vi "Set Serial Settings.vi"(8 "error in (no error)":errorcluster, 11 "LED in":refnum<class "LED.lvclass">) -> (0 "error out":errorcluster, 3 "LED out":refnum<class "LED.lvclass">)   [LabVIEW 2016, in "LED.lvclass"]
uses:
  LED.lvclass
  Desktop/platinum-modbus-driver/omega_engineering-platinum-modbus-driver-671bd10261c3/Labview Source Code/Platinum Serial Modbus/Platinum_MB_SerHandle.ctl
  Desktop/platinum-modbus-driver/omega_engineering-platinum-modbus-driver-671bd10261c3/Labview Source Code/Platinum Serial Modbus/Platinum_MB_serMode.ctl
  Desktop/platinum-modbus-driver/omega_engineering-platinum-modbus-driver-671bd10261c3/Labview Source Code/Platinum Serial Modbus/Platinum_MB_serFlowControl.ctl
  Desktop/platinum-modbus-driver/omega_engineering-platinum-modbus-driver-671bd10261c3/Labview Source Code/Platinum Serial Modbus/Platinum_MB_serParity.ctl
  LED.lvclass/LED.ctl
  LightBox/LightBox.lvclass
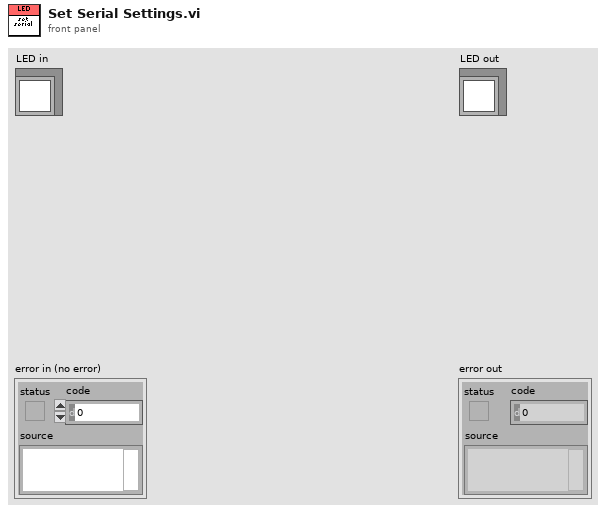
[diagram p1: front panel]
types:
  T1 = typedef "Platinum_MB_serFlowControl.ctl" = enum16{"None", "XON_XOFF", "RTS_CTS", "XON_XOFF_and_RTS_CTS", "DTR_DSR", "XON_XOFF_and_DTR_DSR"}
  T2 = typedef "Platinum_MB_serMode.ctl" = enum16{"RTU", "ASCII"}
  T3 = typedef "Platinum_MB_serParity.ctl" = enum16{"None", "Odd", "Even", "Mark", "Space"}
  T4 = typedef "Platinum_MB_SerHandle.ctl" = cluster{"VISAResourceName":string, "Mode":T2, "Timeout":u32, "FlowControl":T1, "Parity":T3, "BaudRate":u32, "SlaveAddress":u8}
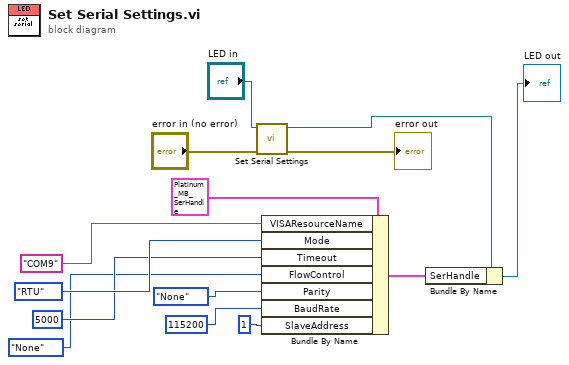
[diagram p0: block diagram]
diagram:
  n1 = call-parent "Set Serial Settings.vi"("error in (no error)"="error in (no error)", "LightBox in"="LED in") -> ("error out"=→"error out":errorcluster, "LightBox out"=w6:refnum<class "LED.lvclass">)  [unwired: 8 in]
  n2 = Bundle By Name(cluster=T4 {"VISAResourceName"="COM9", "Mode"=enum."RTU", "Timeout"=500, "FlowControl"=enum."None", "Parity"=enum."None", "BaudRate"=9600, "SlaveAddress"=1} ("SerHandle"), "VISAResourceName"="COM9", "Mode"=Platinum_MB_serMode."RTU", "Timeout"=u32 5000, "FlowControl"=Platinum_MB_serFlowControl."None", "Parity"=Platinum_MB_serParity."None", "BaudRate"=u32 115200, "SlaveAddress"=u8 1) -> (w10:T4)
  n3 = Bundle By Name(cluster=w6, "SerHandle"=w10) -> (→"LED out":refnum<class "LED.lvclass">)
